vi "Set Ramp Rate Segments.vi"(1 "error in":T2, 2 "Segments":i32=1, 3 "Communications Config":T1={"GPIB address"=22, "GPIB bus"=0, "connection ID"=refnum, "IP"="192.168.2.200", "Active Comm Interface"=0, "Serial Port"="", "Programmer Type"=0} {"Programmer Type" items=["Model 430", "Model 420"]; "Active Comm Interface" items=["TCP/IP (Model 430 Only)", "RS232", "IEEE488"]}) -> (0 "error out":T2)   [LabVIEW 2019]
panel:
  in  "GPIB Address":cluster{"GPIB address":i16, "GPIB bus":i16}={"GPIB address"=22, "GPIB bus"=0}
  out "resulting string":string
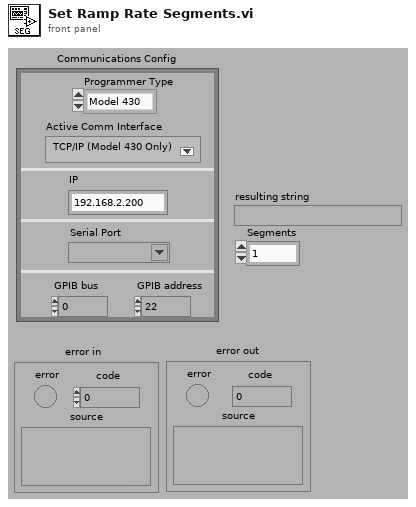
[diagram p1: front panel]
types:
  T1 = cluster{"GPIB address":i16, "GPIB bus":i16, "connection ID":refnum<k5>, "IP":string, "Active Comm Interface":u16, "Serial Port":refnum<visa-resource-name>, "Programmer Type":u16}
  T2 = cluster{"error":bool, "code":i32, "source":string}
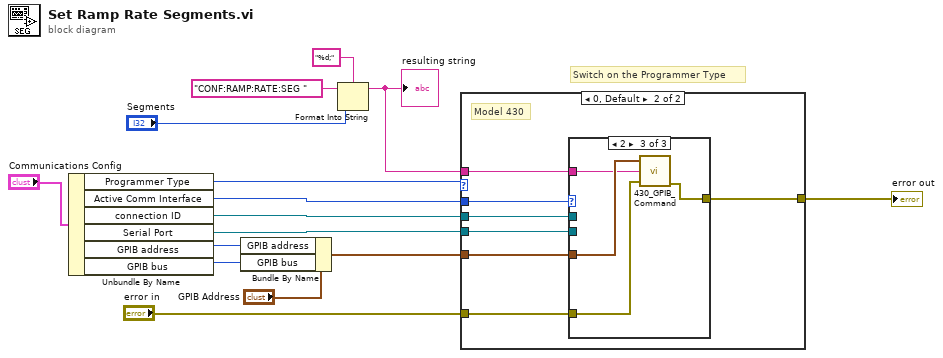
[diagram p0: block diagram]
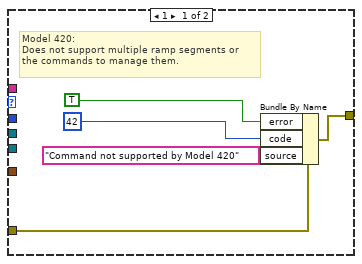
[diagram p2: hidden frame]
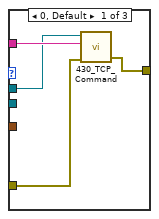
[diagram p3: hidden frame]
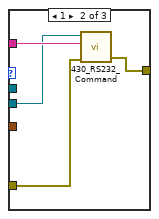
[diagram p4: hidden frame]
diagram:
  # "Switch on the Programmer Type"
  n1 = Unbundle By Name("Communications Config") -> ("Programmer Type"=w1:u16, "Active Comm Interface"=w7:u16, "connection ID"=w8:refnum<k5>, "Serial Port"=w6:refnum<visa-resource-name>, "GPIB address"=w11:i16, "GPIB bus"=w10:i16)
  n2 = Bundle By Name(cluster="GPIB Address", "GPIB address"=w11, "GPIB bus"=w10) -> (w5:cluster{"GPIB address":i16, "GPIB bus":i16})
  n3 = Format Into String(format string="%d;", initial string="CONF:RAMP:RATE:SEG ", "Segments") -> (resulting string=w4:string)  [unwired: 1 in, 1 out]
  "resulting string" <- w4
  n4 = case shown="0, Default" w1 {
    tunnel: w8 -> [_ w27]
    tunnel: w7 -> [_ w26]
    tunnel: w6 -> [_ w25]
    tunnel: w5 -> [_ w24]
    tunnel: w4 -> [_ w23]
    tunnel: [w17 w22] -> w3
    tunnel: "error in" -> [w16 w21]
    frame 1 {
      # "Model 420:\nDoes not support multiple ramp segments or\nthe commands to manage them."
      n5 = Bundle By Name(cluster=w16, "error"=TRUE, "code"=42, "source"="Command not supported by Model 420") -> (w17:T2)
    }
    frame 0, Default {
      # "Model 430"
      n6 = case shown="2" w26 {
        tunnel: w23 -> [w30 w34 w38]
        tunnel: w21 -> [w31 w35 w37]
        tunnel: w25 -> [_ w33 _]
        tunnel: w27 -> [w29 _ _]
        tunnel: w24 -> [_ _ w39]
        tunnel: [w28 w32 w36] -> w22
        frame 0, Default {
          n7 = call "430_TCP_Command.vi"("error in (no error)"=w31, "Command"=w30, "connection ID"=w29) -> ("error out"=w28:errorcluster)  [unwired: 1 in, 2 out]
        }
        frame 1 {
          n8 = call "430_RS232_Command.vi"("error in (no error)"=w35, "Command"=w34, "VISA resource name"=w33) -> ("error out"=w32:errorcluster)  [unwired: 1 in, 2 out]
        }
        frame 2 {
          n9 = call "430_GPIB_Command.vi"("GPIB (In)"=w39, "Input command"=w38, "error in"=w37) -> ("error out"=w36:T2)  [unwired: 3 out]
        }
      }
    }
  }
  "error out" <- w3
